vi "Get All Elements.vi"(3 "Error In":errorcluster, 4 "Delete?":bool, 5 "object in":refnum<class "Stack.lvclass">) -> (0 "Error Out":errorcluster, 1 "Stack Array":variant[](array[variant]), 2 "object out":refnum<class "Stack.lvclass">)   [LabVIEW 2024, in "Stack.lvclass"]
doc: "Return all elements similar to pop."
uses:
  Stack.lvclass
  Stack.lvclass/Stack.ctl
panel:
  # "Connector Pane"
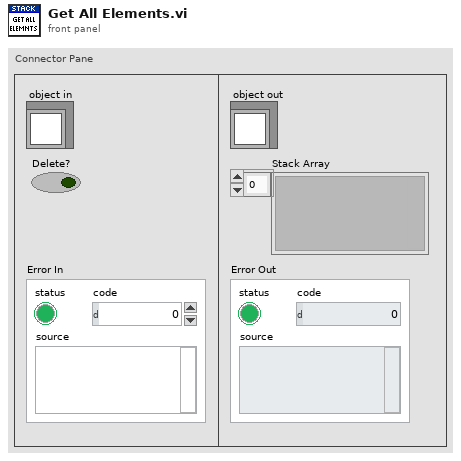
[diagram p1: front panel]
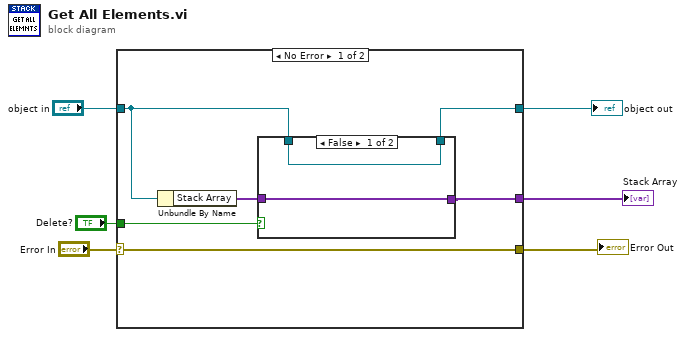
[diagram p0: block diagram]
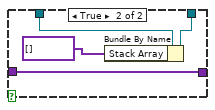
[diagram p2: hidden frame]
diagram:
  n1 = case shown="No Error" "Error In" {
    selector: "Error In" -> [w12 w20]
    tunnel: [w12 w20] -> w5
    tunnel: [w10 w19] -> w3
    tunnel: "object in" -> [w11 w19]
    tunnel: "Delete?" -> [w9 _]
    tunnel: [w7 _] -> w1
    frame No Error {
      n2 = Unbundle By Name(w11) -> ("Stack Array"=w8:variant[])
      n3 = case shown="False" w9 {
        tunnel: w11 -> [w14 w18]
        tunnel: [w14 w17] -> w10
        tunnel: w8 -> [w13 w15]
        tunnel: [w13 w15] -> w7
        frame False {
        }
        frame True {
          n4 = Bundle By Name(cluster=w18, "Stack Array"=variant[] []) -> (w17:refnum<class "Stack.lvclass">)
        }
      }
    }
    frame Error {
    }
  }
  "Error Out" <- w5
  "object out" <- w3
  "Stack Array" <- w1
